vi "intrument_init.vi"(8 "limiting current":dbl, 9 "pld_3605_visa_input":refnum<visa-resource-name>, 11 "keithley_6510_visa_input":refnum<visa-resource-name>) -> (0 "pld_3605_error_output":errorcluster, 1 "pld_3605_visa_output":refnum<visa-resource-name>, 2 "keithley_6510_error_output":errorcluster, 3 "keithley_6510_visa_output":refnum<visa-resource-name>)   [LabVIEW 2019]
uses:
  <vilib>/Instr/_visa.llb/VISA Configure Serial Port (Instr).vi
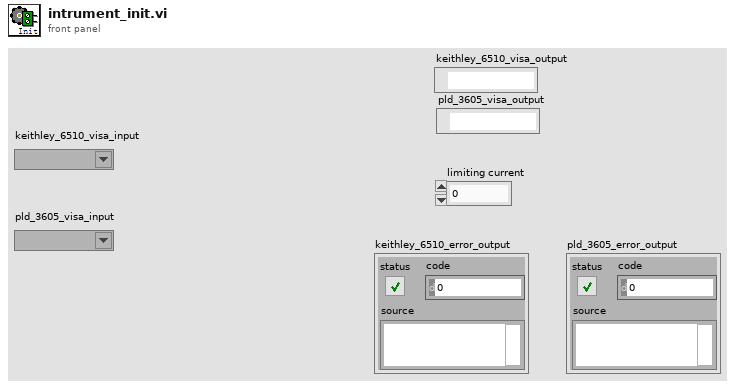
[diagram p1: front panel]
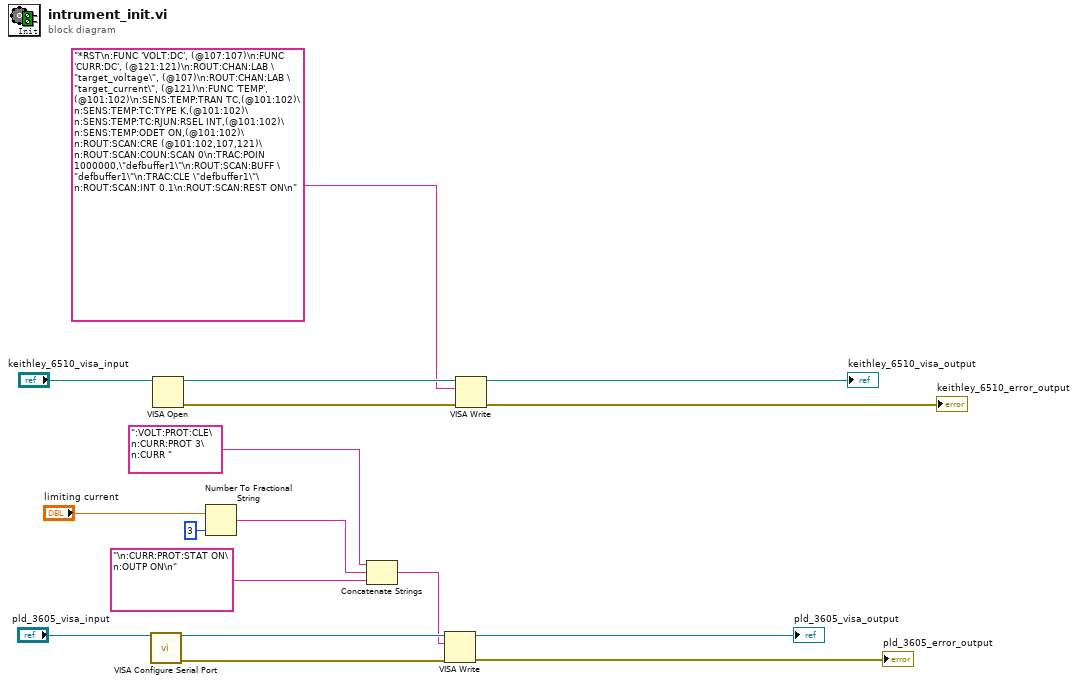
[diagram p0: block diagram]
diagram:
  n1 = call-poly "VISA Configure Serial Port"("VISA resource name"="pld_3605_visa_input") -> ("VISA resource name out"=w12:refnum<visa-resource-name>, "error out"=w11:errorcluster)  [unwired: 13 in]
  n2 = VISA Open(VISA resource name="keithley_6510_visa_input") -> (VISA resource name=w15:refnum<visa-resource-name>, error out=w14:errorcluster)  [unwired: 4 in]
  n3 = Number To Fractional String(number="limiting current", precision (6)=i16 3) -> (F-format string=w4:string)  [unwired: 2 in]
  n4 = Concatenate Strings(":VOLT:PROT:CLE\n:CURR:PROT 3\n:CURR " ("write buffer"), w4, "\n:CURR:PROT:STAT ON\n:OUTP ON\n" ("write buffer")) -> (w1:string)
  n5 = VISA Write(VISA resource name=w12, write buffer=w1, error in (no error)=w11) -> (VISA resource name out=→"pld_3605_visa_output":refnum<visa-resource-name>, error out=→"pld_3605_error_output":errorcluster)  [unwired: 1 out]
  n6 = VISA Write(VISA resource name=w15, write buffer="*RST\n:FUNC 'VOLT:DC', (@107:107)\n:FUNC 'CURR:DC', (@121:121)\n:ROUT:CHAN:LAB \"target_voltage\", (@107)\n:ROUT:CHAN:LAB \"target_current\", (@121)\n:FUNC 'TEMP', (@101:102)\n:SENS:TEMP:TRAN TC,(@101:102)\n:SENS:TEMP:TC:TYPE K,(@101:102)\n:SENS:TEMP:TC:RJUN:RSEL INT,(@101:102)\n:SENS:TEMP:ODET ON,(@101:102)\n:ROUT:SCAN:CRE (@101:102,107,121)\n:ROUT:SCAN:COUN:SCAN 0\n:TRAC:POIN 1000000,\"defbuffer1\"\n:ROUT:SCAN:BUFF \"defbuffer1\"\n:TRAC:CLE \"defbuffer1\"\n:ROUT:SCAN:INT 0.1\n:ROUT:SCAN:REST ON\n", error in (no error)=w14) -> (VISA resource name out=→"keithley_6510_visa_output":refnum<visa-resource-name>, error out=→"keithley_6510_error_output":errorcluster)  [unwired: 1 out]
